vi "Periodic Tasks.vi"() -> ()   [LabVIEW 2011]
doc: "This VI runs in parallel to other tasks. It can contain as many user-defined periodic loops as you need. These can carry out PID or other sorts of timed response."
uses:
  <vilib>/Rock Robotics/SystemInterfaces/Utilities/FPGA_UtilitiesLED State.ctl
  <vilib>/Rock Robotics/SystemInterfaces/Utilities/FPGA_UtilitiesLED Source.ctl
  Robot Global Data.vi
  <vilib>/Rock Robotics/WPI/Relay/WPI_RelayValue.ctl
panel:
  out "Auton Recording":bool
  in  "Turn on Record":bool
  in  "Auton Array":dbl[][](array[numeric])
  out "Ramp ACT Pot":dbl
  in  "Speed of Harvester":dbl
  in  "Speed of Conveyor":dbl
  out "Right Rate":dbl
  out "Right Direction":bool
  out "Right Distance":dbl
  out "Shooter Encoder Distance":dbl
  out "Shooter Direction":bool
  out "Shooter Encoder Rate":dbl
  out "Left Rate":dbl
  out "Gyro Rate":dbl
  out "Gyro Angle":dbl
  out "Left Direction":bool
  out "Left Distance":dbl
  # "Auton Recording"
  # "Sensor Feedback"
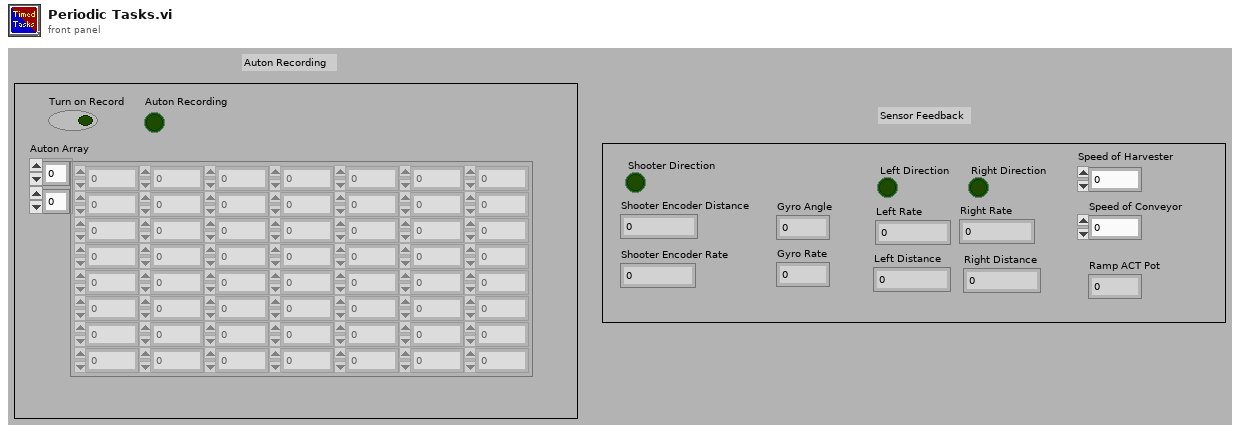
[diagram p1: front panel]
types:
  T1 = typedef "WPI_RelayValue.ctl" = enum16{"Off", "On", "Forward", "Reverse"}
  T2 = typedef "WPI_AnalogChannelDevRef.ctl" = cluster{"DevStatus":errorcluster, "Analog Module":T3, "Analog Channel":T4}
  T3 = typedef "FPGA_TypedefAnalogModule.ctl" = enum16{"Analog Module 1", "Analog Module 2"}
  T4 = typedef "FPGA_AIChannel.ctl" = enum8{"AI 1", "AI 2", "AI 3", "AI 4", "AI 5", "AI 6", "AI 7", "AI 8", "Invalid"}
  T5 = typedef "WPI_EncoderDevRef.ctl" = cluster{"DevStatus":errorcluster, "EncoderIndex":T6, "CounterIndex":T7, "DistancePerCount":dbl, "Decoding Type":T8}
  T6 = typedef "FPGA_EncoderIdx.ctl" = enum8{"Enc 0", "Enc 1", "Enc 2", "Enc 3", "Invalid"}
  T7 = typedef "FPGA_CounterCtrSystemIndex.ctl" = enum8{"Ctr 0", "Ctr 1", "Ctr 2", "Ctr 3", "Ctr 4", "Ctr 5", "Ctr 6", "Ctr 7", "Invalid"}
  T8 = typedef "WPI_EncoderType.ctl" = enum16{"1x", "2x", "4x"}
  T9 = typedef "WPI_GyroDevRef.ctl" = cluster{"DevStatus":errorcluster, "Analog Module":T3, "Analog Channel":T4, "Offset":dbl, "Gain (VoltsPerDegree/Second)":dbl}
  T10 = typedef "WPI_RelayDevRef.ctl" = cluster{"DevStatus":errorcluster, "Relay Channel":T11, "Digital Module":T12, "Relay Direction":T13}
  T11 = typedef "FPGA_DIORelayChannel.ctl" = enum8{"Relay 1", "Relay 2", "Relay 3", "Relay 4", "Relay 5", "Relay 6", "Relay 7", "Relay 8", "Invalid"}
  T12 = typedef "FPGA_TypedefDigitalModule.ctl" = enum16{"Digital Module 1", "Digital Module 2"}
  T13 = typedef "WPI_RelayDirection.ctl" = enum16{"Both directions", "Forward only", "Reverse only"}
  T14 = typedef "FPGA_UtilitiesLED State.ctl" = enum16{"Off", "On", "Toggle"}
  T15 = typedef "FPGA_UtilitiesLED Source.ctl" = enum16{"User LED", "FPGA LED"}
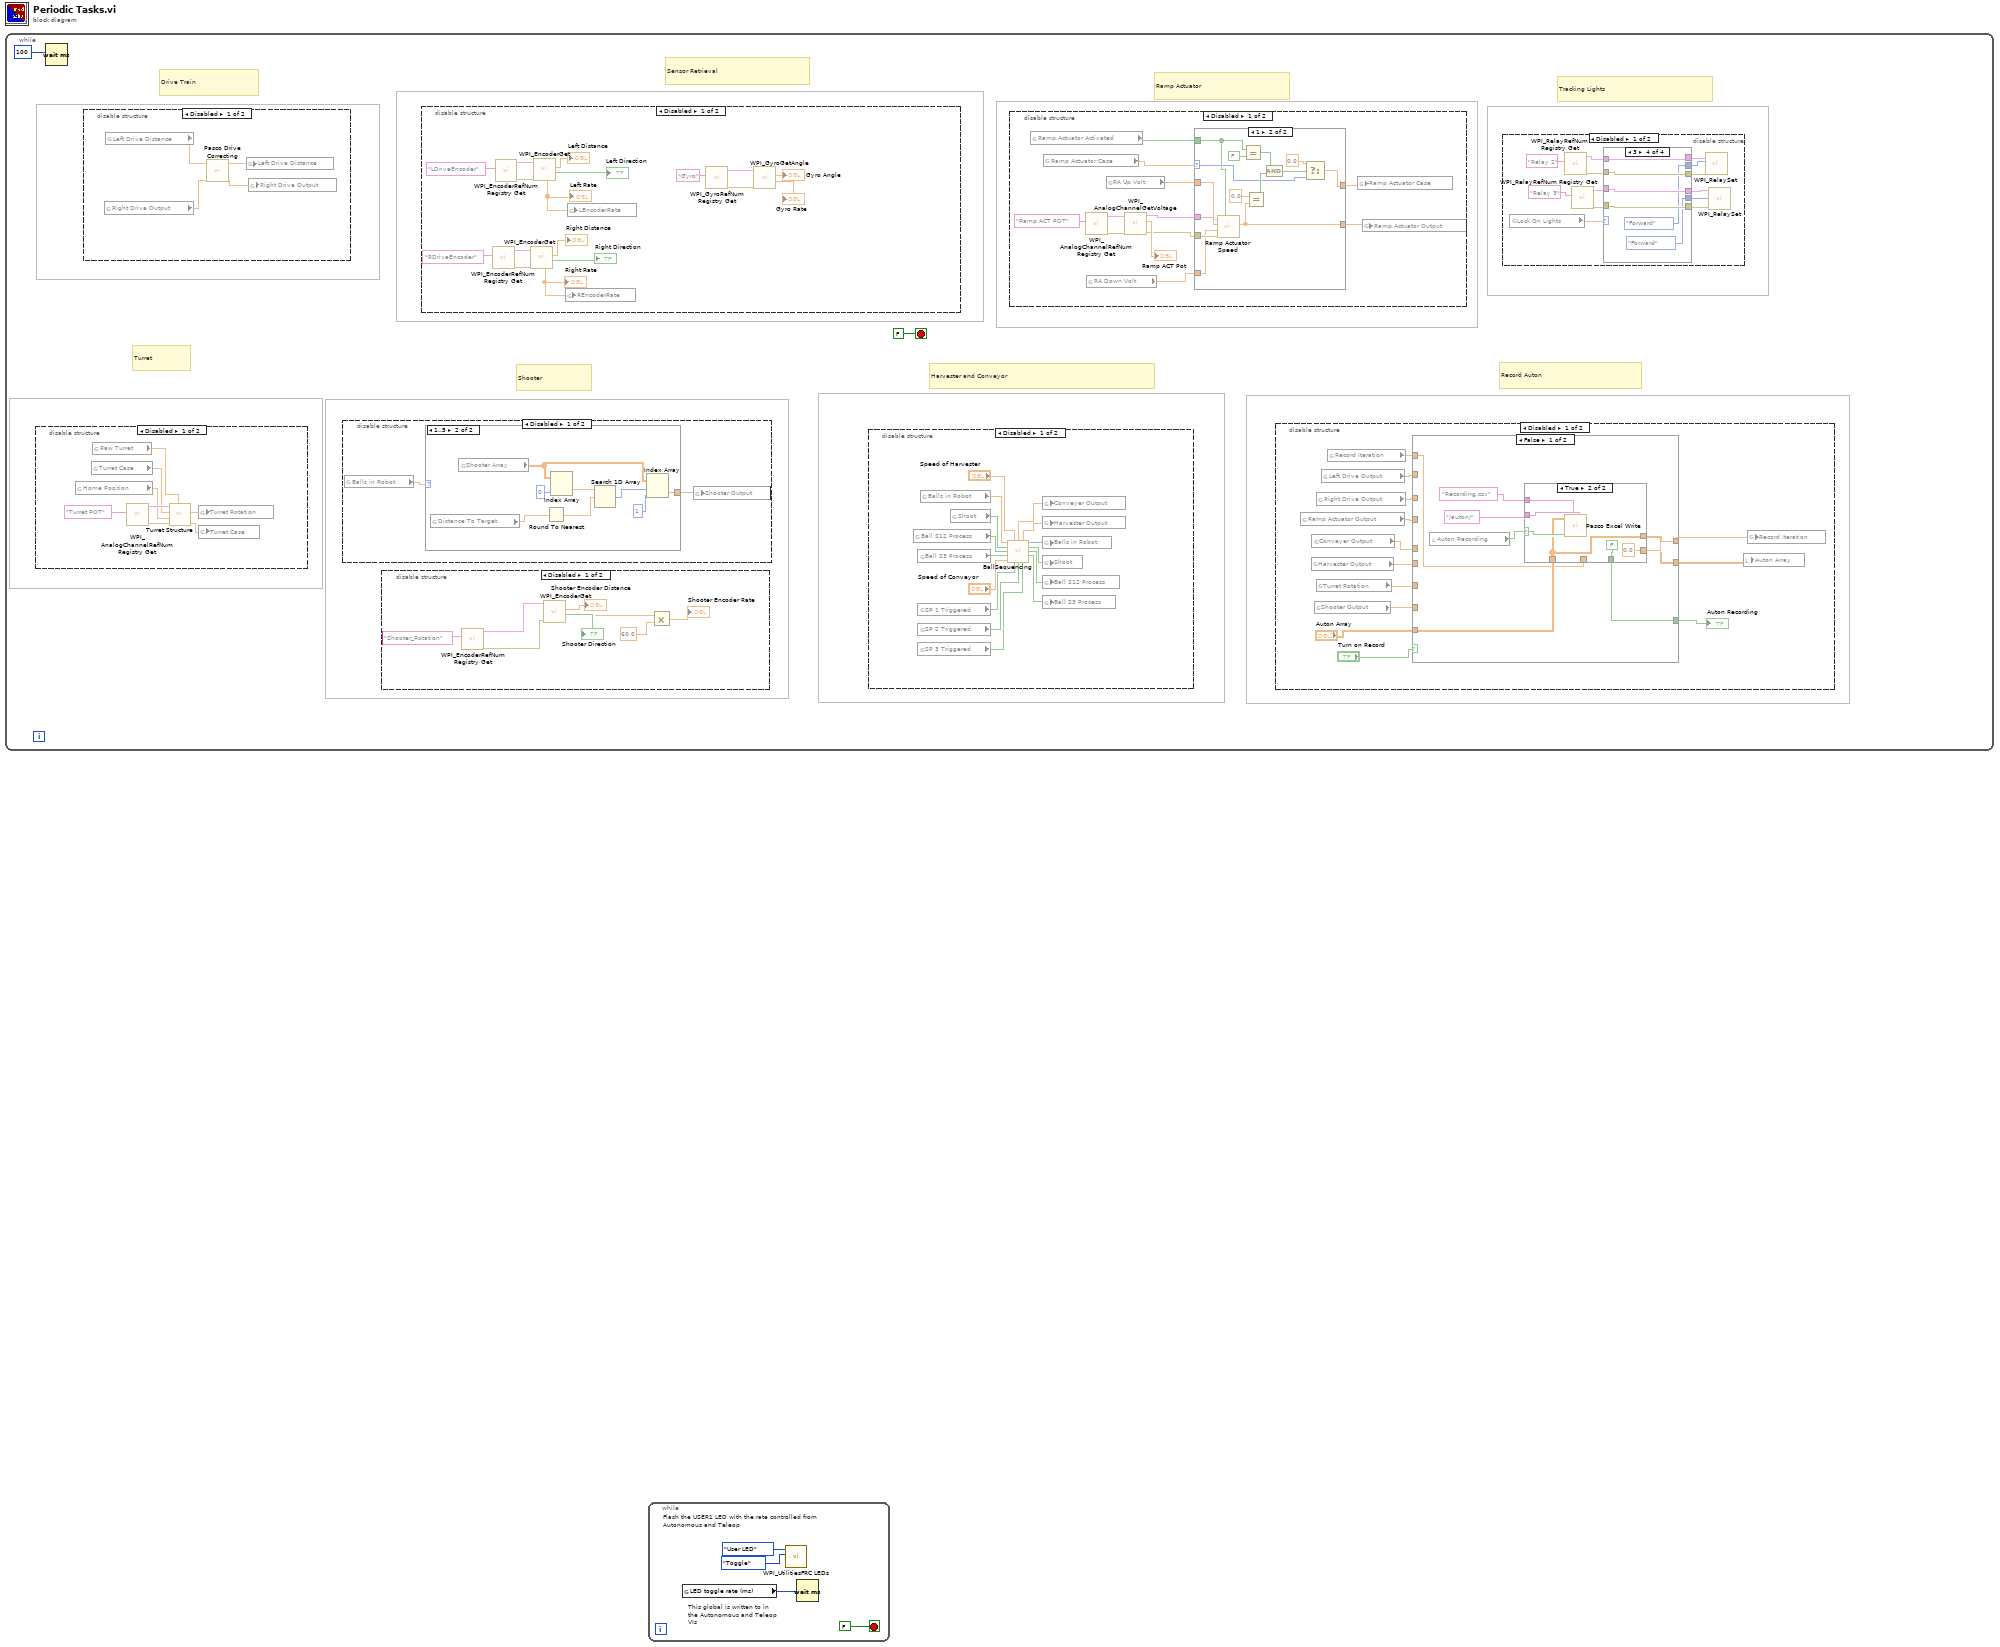
[diagram p0: block diagram]
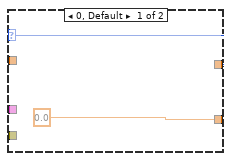
[diagram p3: hidden frame]
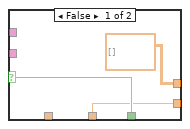
[diagram p5: hidden frame]
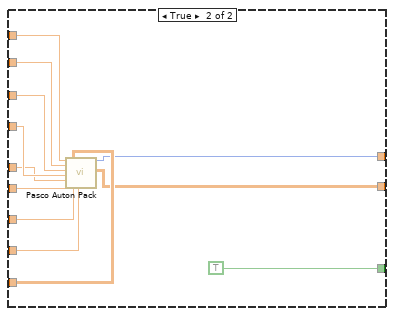
[diagram p6: hidden frame]
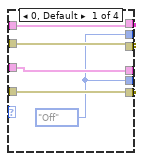
[diagram p8: hidden frame]
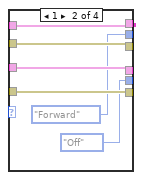
[diagram p9: hidden frame]
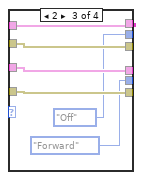
[diagram p10: hidden frame]
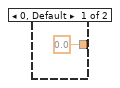
[diagram p12: hidden frame]
diagram:
  n1 = while {
    stop <- FALSE stop-if-true
    # "Tracking Lights"
    # "Record Auton"
    # "Harvester and Conveyor"
    # "Shooter"
    # "Sensor Retrieval"
    # "Turret"
    # "Drive Train"
    # "Ramp Actuator"
    n2 = disable-structure shown="Disabled" {
      frame Disabled {
        n3 = global read "Robot Global Data.vi" "Home Position"() -> (w155:dbl)
        n4 = global read "Robot Global Data.vi" "Turret Case"() -> (w156:dbl)
        n5 = global read "Robot Global Data.vi" "Raw Turret"() -> (w154:dbl)
        n6 = call <vilib>:"WPI_AnalogChannelRefNum Registry Get.vi"("refnum name"="Turret POT") -> ("error out"=w157:errorcluster, "AIDeviceRef"=w158:T2)  [unwired: 9 in]
        n7 = call "Turret Structure.vi"("Raw Turret"=w154, "error in (no error)"=w157, "Home postion"=w155, "Turret Case"=w156, "AIDeviceRef"=w158) -> ("Turret Case Output"=w152:dbl, "Turret Output"=w153:dbl)  [unwired: 5 in]
        n8 = global write "Robot Global Data.vi" "Turret Rotation"(w153) -> ()
        n9 = global write "Robot Global Data.vi" "Turret Case"(w152) -> ()
      }
      frame Enabled {
      }
    }
    n10 = Wait (ms)(milliseconds to wait=u32 100) -> ()  [unwired: 1 out]
    n11 = disable-structure shown="Disabled" {
      frame Disabled {
        n12 = global read "Robot Global Data.vi" "Right Drive Output"() -> (w162:dbl)
        n13 = global read "Robot Global Data.vi" "Left Drive Distance"() -> (w163:dbl)
        n14 = call "Pasco Drive Correcting.vi"("RightDriveOutput"=w162, "LeftDriveOutput"=w163) -> ("RightDriveOutput"=w160:dbl, "LeftDriveOutput"=w161:dbl)  [unwired: 8 in]
        n15 = global write "Robot Global Data.vi" "Left Drive Distance"(w161) -> ()
        n16 = global write "Robot Global Data.vi" "Right Drive Output"(w160) -> ()
      }
      frame Enabled {
      }
    }
    n17 = disable-structure shown="Disabled" {
      frame Disabled {
        n18 = global read "Robot Global Data.vi" "Balls in Robot"() -> (w126:dbl)
        n19 = case shown="1..5" w126 {
          tunnel: [0.0 w131] -> w127
          frame 0, Default {
          }
          frame 1..5 {
            n20 = global read "Robot Global Data.vi" "Distance To Target"() -> (w130:dbl)
            n21 = global read "Robot Global Data.vi" "Shooter Array"() -> (w134:dbl[][])
            n22 = Round To Nearest(number=w130) -> (nearest integer value=w129:dbl)
            n23 = Index Array(array=w134, index (col)=0 ("disabled index (col)")) -> (element=w135:dbl[])  [unwired: 1 in]
            n24 = Search 1D Array(1D array=w135, element=w129) -> (index of element=w133:i32)  [unwired: 1 in]
            n25 = Index Array(array=w134, index (row)=w133, index (col)=1 ("disabled index (col)")) -> (element=w131:dbl)
          }
        }
        n26 = global write "Robot Global Data.vi" "Shooter Output"(w127) -> ()
      }
      frame Enabled {
      }
    }
    n27 = disable-structure shown="Disabled" {
      frame Disabled {
        n28 = call <vilib>:"WPI_EncoderRefNum Registry Get.vi"("refnum name"="Shooter_Rotation") -> ("error out"=w164:errorcluster, "EncoderDevRef"=w165:T5)  [unwired: 9 in]
        n29 = call <vilib>:"WPI_EncoderGet.vi"("error in (no error)"=w164, "EncoderDevRef"=w165) -> ("Direction"=→"Shooter Direction":bool, "Distance"=→"Shooter Encoder Distance":dbl, "Rate"=w168:dbl)  [unwired: 4 in, 3 out]
        n30 = Multiply(x=w168, y=60.0) -> (x*y=→"Shooter Encoder Rate":dbl)
      }
      frame Enabled {
      }
    }
    n31 = disable-structure shown="Disabled" {
      frame Disabled {
        n32 = call <vilib>:"WPI_EncoderRefNum Registry Get.vi"("refnum name"="RDriveEncoder") -> ("error out"=w12:errorcluster, "EncoderDevRef"=w11:T5)  [unwired: 9 in]
        n33 = call <vilib>:"WPI_EncoderRefNum Registry Get.vi"("refnum name"="LDriveEncoder") -> ("error out"=w18:errorcluster, "EncoderDevRef"=w17:T5)  [unwired: 9 in]
        n34 = call <vilib>:"WPI_EncoderGet.vi"("error in (no error)"=w12, "EncoderDevRef"=w11) -> ("Direction"=→"Right Direction":bool, "Distance"=→"Right Distance":dbl, "Rate"=w8:dbl)  [unwired: 4 in, 3 out]
        "Right Rate" <- w8
        n35 = call <vilib>:"WPI_EncoderGet.vi"("error in (no error)"=w18, "EncoderDevRef"=w17) -> ("Direction"=→"Left Direction":bool, "Distance"=→"Left Distance":dbl, "Rate"=w14:dbl)  [unwired: 4 in, 3 out]
        "Left Rate" <- w14
        n36 = global write "Robot Global Data.vi" "REncoderRate"(w8) -> ()
        n37 = global write "Robot Global Data.vi" "LEncoderRate"(w14) -> ()
        n38 = call <vilib>:"WPI_GyroRefNum Registry Get.vi"("refnum name"="Gyro") -> ("error out"=w6:errorcluster, "GyroDevRef"=w7:T9)  [unwired: 9 in]
        n39 = call <vilib>:"WPI_GyroGetAngle.vi"("error in (no error)"=w6, "GyroDevRef"=w7) -> ("Angular Rate"=→"Gyro Rate":dbl, "Angle"=→"Gyro Angle":dbl)  [unwired: 6 in, 2 out]
      }
      frame Enabled {
      }
    }
    n40 = disable-structure shown="Disabled" {
      frame Disabled {
        n41 = global read "Robot Global Data.vi" "Ball S12 Process"() -> (w138:bool)
        n42 = global read "Robot Global Data.vi" "Ball S3 Process"() -> (w137:bool)
        n43 = global read "Robot Global Data.vi" "SP 1 Triggered"() -> (w145:bool)
        n44 = global read "Robot Global Data.vi" "SP 2 Triggered"() -> (w146:bool)
        n45 = global read "Robot Global Data.vi" "SP 3 Triggered"() -> (w147:bool)
        n46 = global read "Robot Global Data.vi" "Balls in Robot"() -> (w140:dbl)
        n47 = global read "Robot Global Data.vi" "Shoot"() -> (w139:bool)
        n48 = call "BallSequencing.vi"("Balls In Robot"=w140, "Speed of Harvester"="Speed of Harvester", "Shoot"=w139, "Ball S12 Process"=w138, "Ball S3 Process"=w137, "Speed of Conveyor"="Speed of Conveyor", "SP 1 Triggered"=w145, "SP 2 Triggered"=w146, "SP 3 Triggered"=w147) -> ("Conveyer Output"=w141:dbl, "Harvester Output"=w142:dbl, "Balls In Robot Output"=w151:i32, "Shoot Output"=w150:bool, "Ball S12 Process Output"=w149:bool, "Ball S3 Process Output"=w148:bool)  [unwired: 1 in]
        n49 = global write "Robot Global Data.vi" "Conveyer Output"(w141) -> ()
        n50 = global write "Robot Global Data.vi" "Harvester Output"(w142) -> ()
        n51 = global write "Robot Global Data.vi" "Balls in Robot"(w151) -> ()
        n52 = global write "Robot Global Data.vi" "Shoot"(w150) -> ()
        n53 = global write "Robot Global Data.vi" "Ball S12 Process"(w149) -> ()
        n54 = global write "Robot Global Data.vi" "Ball S3 Process"(w148) -> ()
      }
      frame Enabled {
      }
    }
    n55 = disable-structure shown="Disabled" {
      frame Disabled {
        n56 = global read "Robot Global Data.vi" "Ramp Actuator Activated"() -> (w25:bool)
        n57 = global read "Robot Global Data.vi" "Ramp Actuator Case"() -> (w27:dbl)
        n58 = call <vilib>:"WPI_AnalogChannelRefNum Registry Get.vi"("refnum name"="Ramp ACT POT") -> ("error out"=w23:errorcluster, "AIDeviceRef"=w24:T2)  [unwired: 9 in]
        n59 = global read "Robot Global Data.vi" "RA Down Volt"() -> (w30:dbl)
        n60 = global read "Robot Global Data.vi" "RA Up Volt"() -> (w29:dbl)
        n61 = call <vilib>:"WPI_AnalogChannelGetVoltage.vi"("error in (no error)"=w23, "AIDeviceRef"=w24) -> ("error out"=w20:errorcluster, "Voltage"=→"Ramp ACT Pot":dbl, "AIDeviceRef"=w21:T2)  [unwired: 7 in]
        n62 = case shown="1" w27 {
          selector: w27 -> [w32 w37]
          tunnel: w20 -> [_ w47]
          tunnel: w30 -> [_ w46]
          tunnel: w29 -> [_ w45]
          tunnel: [0.0 ("Ramp Actuator Ouput") w36] -> w28
          tunnel: w25 -> [_ w35]
          tunnel: [w32 w38] -> w26
          tunnel: w21 -> [_ w34]
          frame 0, Default {
          }
          frame 1 {
            n63 = call "Ramp Actuator Speed.vi"("Up to Down"=w35, "error in (no error)"=w47, "RA Down Volt"=w46, "RA Up Volt"=w45, "AIDeviceRef"=w34) -> ("Ramp Actuator Ouput"=w36:dbl)  [unwired: 6 in]
            n64 = Equal?(x=w35, y=FALSE) -> (x = y?=w42:bool)
            n65 = Equal?(x=0.0, y=w36) -> (x = y?=w43:bool)
            n66 = And(x=w42, y=w43) -> (x .and. y?=w40:bool)
            n67 = Select(t=0.0, s=w40, f=w37) -> (s? t:f=w38:dbl)
          }
        }
        n68 = global write "Robot Global Data.vi" "Ramp Actuator Case"(w26) -> ()
        n69 = global write "Robot Global Data.vi" "Ramp Actuator Output"(w28) -> ()
      }
      frame Enabled {
      }
    }
    n70 = disable-structure shown="Disabled" {
      frame Disabled {
        n71 = global read "Robot Global Data.vi" "Ramp Actuator Output"() -> (w57:dbl)
        n72 = global read "Robot Global Data.vi" "Harvester Output"() -> (w55:dbl)
        n73 = global read "Robot Global Data.vi" "Conveyer Output"() -> (w56:dbl)
        n74 = global read "Robot Global Data.vi" "Shooter Output"() -> (w53:dbl)
        n75 = global read "Robot Global Data.vi" "Turret Rotation"() -> (w54:dbl)
        n76 = global read "Robot Global Data.vi" "Right Drive Output"() -> (w58:dbl)
        n77 = global read "Robot Global Data.vi" "Left Drive Output"() -> (w59:dbl)
        n78 = global read "Robot Global Data.vi" "Record Iteration"() -> (w60:dbl)
        n79 = case shown="False" "Turn on Record" {
          tunnel: w60 -> [w64 w89]
          tunnel: w59 -> [_ w88]
          tunnel: w58 -> [_ w87]
          tunnel: w57 -> [_ w86]
          tunnel: w56 -> [_ w85]
          tunnel: w55 -> [_ w84]
          tunnel: w54 -> [_ w83]
          tunnel: w53 -> [_ w82]
          tunnel: "Auton Array" -> [w65 w81]
          tunnel: [w61 w80] -> w50
          tunnel: [w62 w79] -> w49
          tunnel: [w63 TRUE] -> w48
          frame False {
            n80 = local read "Auton Recording"() -> (w66:bool)
            n81 = case shown="True" w66 {
              selector: w66 -> [w71 w76]
              tunnel: [w71 FALSE] -> w63
              tunnel: "/auton/" ("File Name") -> [_ w75]
              tunnel: "Recording.csv" ("Folder Location") -> [_ w74]
              tunnel: [w70 0.0 ("Record Iteration")] -> w62
              tunnel: w64 -> [w70 _]
              tunnel: w65 -> [_ w72]
              tunnel: [dbl[][] [] ("Auton Array") w72] -> w61
              frame False {
              }
              frame True {
                n82 = call "Pasco Excel Write.vi"("Folder Location"=w75, "File Name"=w74, "WriteToExcel"=w76, "2D data"=w72) -> ()  [unwired: 7 in, 1 out]
              }
            }
          }
          frame True {
            n83 = call "Pasco Auton Pack.vi"("Iterations"=w89, "Left Drive"=w88, "Right Drive"=w87, "RAMP ACT"=w86, "Conveyor"=w85, "Harvestor"=w84, "Auton Array"=w81, "Turret"=w83, "Shooter"=w82) -> ("Iteration Output"=w79:i32, "output array"=w80:dbl[][])  [unwired: 9 in]
          }
        }
        "Auton Recording" <- w48
        n84 = local write "Auton Array"(w50) -> ()
        n85 = global write "Robot Global Data.vi" "Record Iteration"(w49) -> ()
      }
      frame Enabled {
      }
    }
    n86 = disable-structure shown="Disabled" {
      frame Disabled {
        n87 = global read "Robot Global Data.vi" "Lock On Lights"() -> (w90:dbl)
        n88 = call <vilib>:"WPI_RelayRefNum Registry Get.vi"("refnum name"="Relay 2") -> ("error out"=w97:errorcluster, "RelayDevRef"=w99:T10)  [unwired: 9 in]
        n89 = call <vilib>:"WPI_RelayRefNum Registry Get.vi"("refnum name"="Relay 3") -> ("error out"=w94:errorcluster, "RelayDevRef"=w95:T10)  [unwired: 9 in]
        n90 = case shown="3" w90 {
          tunnel: [w107 w113 w119 w125] -> w100
          tunnel: w99 -> [w107 w113 w119 w125]
          tunnel: [w106 w112 w118 w124] -> w98
          tunnel: w97 -> [w106 w112 w118 w124]
          tunnel: [w105 w111 w117 w123] -> w96
          tunnel: w95 -> [w105 w111 w117 w123]
          tunnel: w94 -> [w104 w110 w116 w122]
          tunnel: [w104 w110 w116 w122] -> w93
          tunnel: [w103 WPI_RelayValue."Forward" ("RelayValue") WPI_RelayValue."Off" ("RelayValue") WPI_RelayValue."Forward" ("RelayValue")] -> w92
          tunnel: [w103 WPI_RelayValue."Off" ("RelayValue") WPI_RelayValue."Forward" ("RelayValue") WPI_RelayValue."Forward" ("RelayValue")] -> w91
          frame 0, Default {
            w103 = WPI_RelayValue."Off" ("RelayValue")
          }
          frame 1 {
          }
          frame 2 {
          }
          frame 3 {
          }
        }
        n91 = call <vilib>:"WPI_RelaySet.vi"("error in (no error)"=w98, "RelayValue"=w92, "RelayDevRef"=w100) -> ()  [unwired: 7 in, 2 out]
        n92 = call <vilib>:"WPI_RelaySet.vi"("error in (no error)"=w93, "RelayValue"=w91, "RelayDevRef"=w96) -> ()  [unwired: 7 in, 2 out]
      }
      frame Enabled {
      }
    }
  }
  n93 = while {
    stop <- FALSE stop-if-true
    # "This global is written to in the Autonomous and Teleop VIs"
    # "Flash the USER1 LED with the rate controlled from Autonomous and Teleop"
    n94 = global read "Robot Global Data.vi" "LED toggle rate (ms)"() -> (w172:u32)
    n95 = call <vilib>:"WPI_UtilitiesFRC LEDs.vi"("State"=FPGA_UtilitiesLED_State."Toggle", "LED Type"=FPGA_UtilitiesLED_Source."User LED") -> ()  [unwired: 1 in, 9 out]
    n96 = Wait (ms)(milliseconds to wait=w172) -> ()  [unwired: 1 out]
  }
